vi "Manual Mode.vi"(5 "slider shoot":dbl, 7 "Shooter":T1, 8 "engage shoot":bool, 9 "Potent":dbl, 11 "Button 1":bool) -> ()   [LabVIEW 2012]
uses:
  <vilib>/Rock Robotics/WPI/Solenoid/WPI_SolenoidValue.ctl
  <vilib>/Rock Robotics/WPI/Joystick/WPI_JoystickGetSetRefNum.vi
  <vilib>/Rock Robotics/WPI/RobotDrive/WPI_RobotDriveArcadeDrive_Standard(NoSaturation).vi
  <vilib>/Rock Robotics/WPI/RobotDrive/WPI_RobotDriveGetSetRefNum.vi
  <vilib>/Rock Robotics/WPI/Solenoid/WPI_SolenoidSetEnum.vi
panel:
  out "theoretical angle":dbl
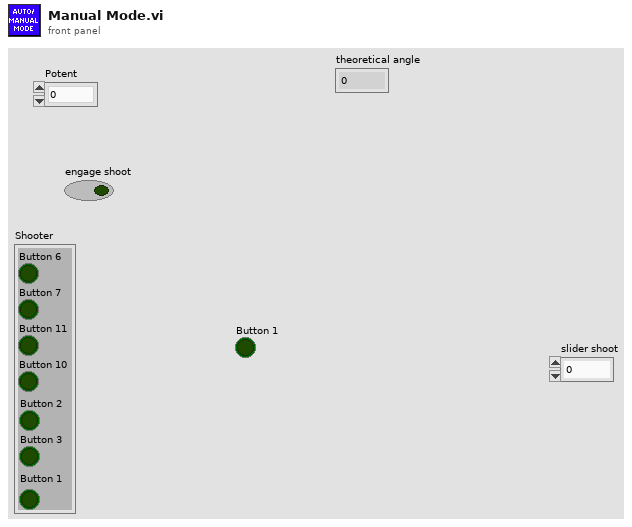
[diagram p1: front panel]
types:
  T1 = cluster{"Button 6":bool, "Button 7":bool, "Button 11":bool, "Button 10":bool, "Button 2":bool, "Button 3":bool, "Button 1":bool}
  T2 = typedef "WPI_JoystickDevRef.ctl" = cluster{"Device":T3}
  T3 = typedef "WPI_JoystickDeviceEnum.ctl" = enum16{"USB 1", "USB 2", "USB 3", "USB 4", "Kinect 1", "Kinect 2"}
  T4 = typedef "WPI_JoystickButtonState.ctl" = cluster{"Button 1":bool, "Button 2":bool, "Button 3":bool, "Button 4":bool, "Button 5":bool, "Button 6":bool, "Button 7":bool, "Button 8":bool, "Button 9":bool, "Button 10":bool, "Button 11":bool, "Button 12":bool}
  T5 = typedef "WPI_SolenoidDevRef.ctl" = cluster{"DevStatus":errorcluster, "Solenoid Module":T6, "Forward Solenoid Channel":T7, "Reverse Solenoid Channel":T7}
  T6 = typedef "FPGA_TypedefSolenoidModule.ctl" = enum16{"Solenoid Module 1", "Solenoid Module 2"}
  T7 = typedef "WPI_SolenoidChannel.ctl" = enum8{"Solenoid 1", "Solenoid 2", "Solenoid 3", "Solenoid 4", "Solenoid 5", "Solenoid 6", "Solenoid 7", "Solenoid 8", "Invalid"}
  T8 = typedef "WPI_MotorControlDeviceRef.ctl" = cluster{"DeviceStatus":errorcluster, "Type":enum16{"PWM", "CAN"}, "PWM":cluster{"Digital Module":T9, "PWM Channel":T10, "DeadBand":T11}, "CAN":cluster{"Device Number":u8, "Control Mode":T12, "Semaphore":T13, "Max Vout":dbl}, "Invert":bool, "TransformRef":T14, "InvTransformRef":T14}
  T9 = typedef "FPGA_TypedefDigitalModule.ctl" = enum16{"Digital Module 1", "Digital Module 2"}
  T10 = typedef "FPGA_DIOPWMChannel.ctl" = enum8{"PWM 1", "PWM 2", "PWM 3", "PWM 4", "PWM 5", "PWM 6", "PWM 7", "PWM 8", "PWM 9", "PWM 10", "Invalid"}
  T11 = typedef "WPI_PWMDeadband.ctl" = cluster{"Name":string, "maxPositivePwm":i32, "minPositivePwm":i32, "centerPwm":i32, "maxNegativePwm":i32, "minNegativePwm":i32, "angularRange":u16}
  T12 = typedef "WPI_CANJaguar_ControlMode.ctl" = enum8{"Percent VBus", "Current", "Speed", "Position", "Voltage"}
  T13 = typedef "Semaphore RefNum" = refnum<k1>
  T14 = typedef "WPI_PWMTransform_ConPane.ctl" = refnum<vi>
  T15 = typedef "WPI_SolenoidValue.ctl" = enum16{"Off", "On", "Forward", "Reverse"}
  T16 = typedef "WPI_RobotDriveDevRef.ctl" = cluster{"DevStatus":errorcluster, "Motors[]":T8[], "Square Inputs":bool, "Max Output":dbl, "Isochronous":bool}
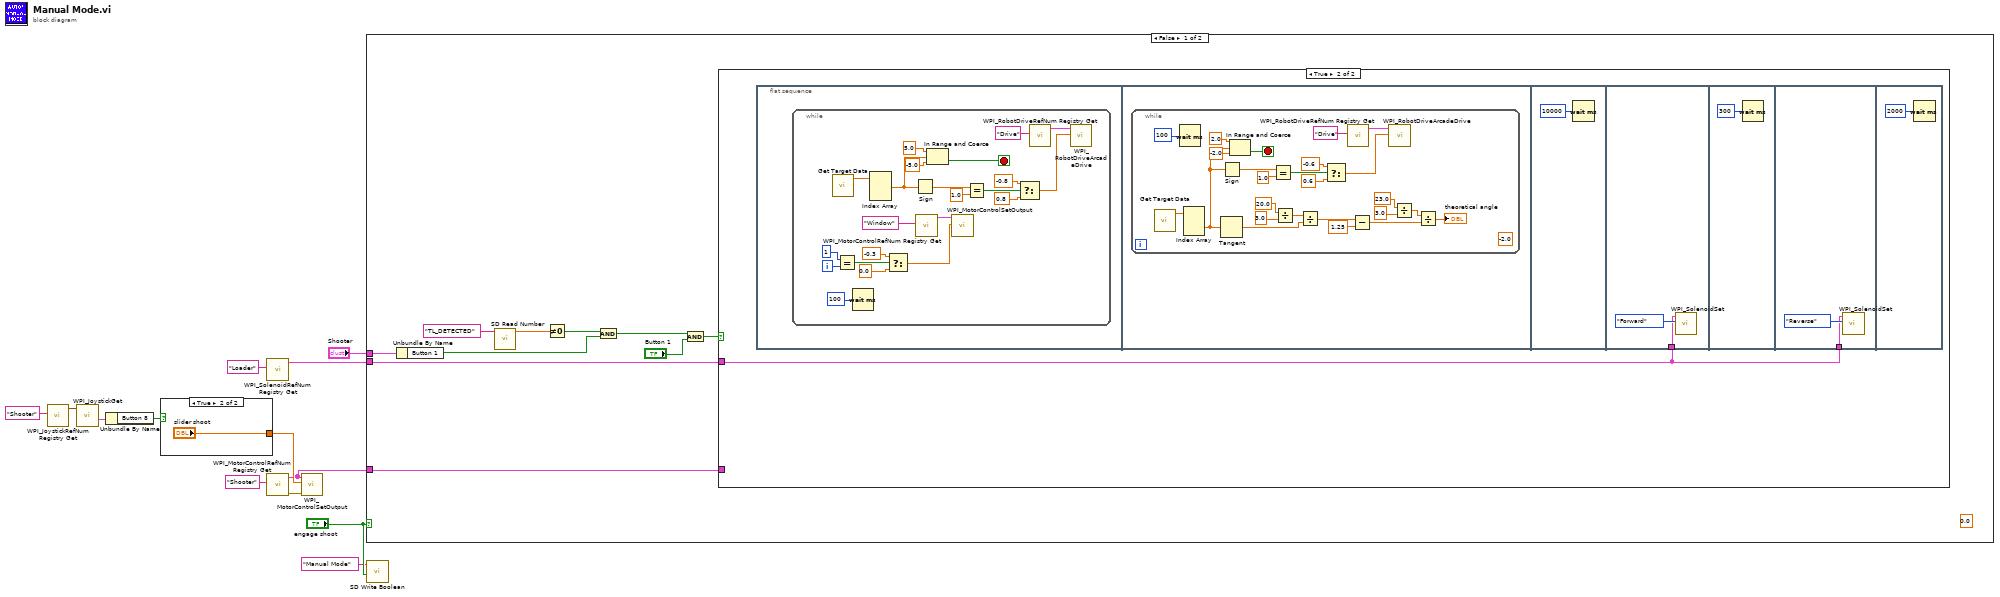
[diagram p0: block diagram]
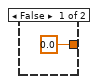
[diagram p2: hidden frame]
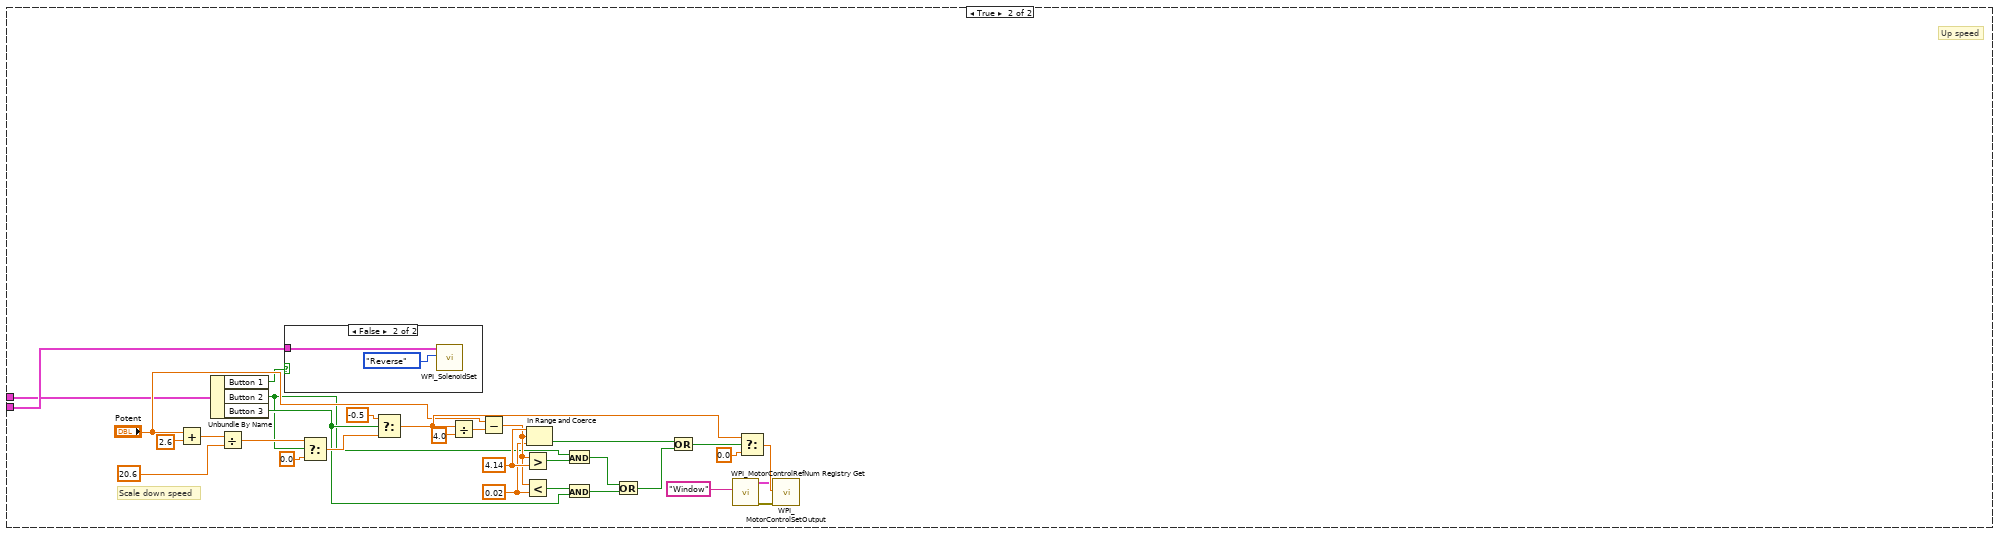
[diagram p4: hidden frame]
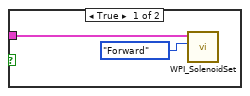
[diagram p5: hidden frame]
diagram:
  n1 = call <vilib>:"WPI_JoystickRefNum Registry Get.vi"("refnum name"="Shooter") -> ("JoystickDevRef"=w3:T2)  [unwired: 9 in, 1 out]
  n2 = call <vilib>:"WPI_JoystickGet.vi"("JoystickDevRef"=w3) -> ("Buttons"=w5:T4)  [unwired: 4 in, 2 out]
  n3 = Unbundle By Name(w5) -> ("Button 8"=w4:bool)
  n4 = case shown="True" w4 {
    tunnel: [0.0 ("slider shoot") "slider shoot"] -> w6
    frame False {
    }
    frame True {
    }
  }
  n5 = call <vilib>:"WPI_SolenoidRefNum Registry Get.vi"("refnum name"="Loader") -> ("SolenoidDevRef"=w11:T5)  [unwired: 9 in, 1 out]
  n6 = call <vilib>:"WPI_MotorControlRefNum Registry Get.vi"("refnum name"="Shooter") -> ("error out"=w8:errorcluster, "MotorControlDevRef"=w1:T8)  [unwired: 9 in]
  n7 = call <vilib>:"WPI_MotorControlSetOutput.vi"("error in (no error)"=w8, "Output"=w6, "MotorControlDevRef"=w1) -> ()  [unwired: 6 in, 3 out]
  n8 = case shown="False" "engage shoot" {
    tunnel: "Shooter" -> [w25 w81]
    tunnel: w11 -> [w22 w82]
    tunnel: w1 -> [w16 _]
    frame False {
      (unwired) 0.0 ("speed")
      n9 = Unbundle By Name(w25) -> ("Button 1"=w21:bool)
      n10 = call <vilib>:"SD Read Number.vi"("Name"="TL_DETECTED") -> ("Numeric"=w17:dbl)  [unwired: 8 in, 2 out]
      n11 = Not Equal To 0?(x=w17) -> (x != 0?=w18:bool)
      n12 = And(x=w18, y=w21) -> (x .and. y?=w20:bool)
      n13 = And(x=w20, y="Button 1") -> (x .and. y?=w24:bool)
      n14 = case shown="True" w24 {
        tunnel: w22 -> [_ w26]
        tunnel: w16 -> [_ _]
        frame False {
        }
        frame True {
          n15 = flat-sequence {
            tunnel: w26 -> [w75]
            tunnel: w26 -> [w78]
            frame #0 {
              n16 = while {
                i -> [w42]
                stop <- w27 stop-if-true
                n17 = call "Get Target Data.vi"() -> ("values"=w29:dbl[])  [unwired: 10 in, 1 out]
                n18 = Equal?(x=1, y=w42) -> (x = y?=w43:bool)
                n19 = Wait (ms)(milliseconds to wait=u32 100) -> ()  [unwired: 1 out]
                n20 = Index Array(array=w29) -> (element #1=w28:dbl)  [unwired: 3 in, 2 out]
                n21 = Select(t=-0.3, s=w43, f=0.0) -> (s? t:f=w40:dbl)
                n22 = Sign(1:w28) -> (0:w34:dbl)
                n23 = call <vilib>:"WPI_MotorControlRefNum Registry Get.vi"("refnum name"="Window") -> ("MotorControlDevRef"=w45:T8)  [unwired: 9 in, 1 out]
                n24 = In Range and Coerce(upper limit=5.0, x=w28, lower limit=-5.0) -> (In Range?=w27:bool)  [unwired: 1 out]
                n25 = call <vilib>:"WPI_MotorControlSetOutput.vi"("Output"=w40, "MotorControlDevRef"=w45) -> ()  [unwired: 7 in, 3 out]
                n26 = Equal?(x=w34, y=1.0) -> (x = y?=w33:bool)
                n27 = Select(t=-0.8, s=w33, f=0.8) -> (s? t:f=w30:dbl)
                n28 = call <vilib>:"WPI_RobotDriveRefNum Registry Get.vi"("refnum name"="Drive") -> ("RobotDriveDevRef"=w47:T16)  [unwired: 9 in, 1 out]
                n29 = call-poly <vilib>:"WPI_RobotDriveArcadeDrive.vi"("X axis value"=w30, "RobotDriveDevRef"=w47) -> ()  [unwired: 7 in, 3 out]
              }
            }
            frame #1 {
              n30 = while {
                stop <- w51 stop-if-true
                (unwired) -2.0 ("lower limit")
                n31 = call "Get Target Data.vi"() -> ("values"=w53:dbl[])  [unwired: 10 in, 1 out]
                n32 = Wait (ms)(milliseconds to wait=u32 100) -> ()  [unwired: 1 out]
                n33 = Index Array(array=w53) -> (element #2=w52:dbl)  [unwired: 3 in, 2 out]
                n34 = Sign(1:w52) -> (0:w56:dbl)
                n35 = Tangent(1:w52) -> (0:w63:dbl)
                n36 = In Range and Coerce(upper limit=2.0, x=w52, lower limit=-2.0) -> (In Range?=w51:bool)  [unwired: 1 out]
                n37 = Equal?(x=w56, y=1.0) -> (x = y?=w55:bool)
                n38 = Divide(x=20.0, y=3.0) -> (x/y=w70:dbl)
                n39 = Divide(x=w70, y=w63) -> (x/y=w64:dbl)
                n40 = Select(t=-0.6, s=w55, f=0.6) -> (s? t:f=w50:dbl)
                n41 = call <vilib>:"WPI_RobotDriveRefNum Registry Get.vi"("refnum name"="Drive") -> ("RobotDriveDevRef"=w72:T16)  [unwired: 9 in, 1 out]
                n42 = Subtract(x=w64, y=1.25) -> (x-y=w66:dbl)
                n43 = call-poly <vilib>:"WPI_RobotDriveArcadeDrive.vi"("X axis value"=w50, "RobotDriveDevRef"=w72) -> ()  [unwired: 7 in, 3 out]
                n44 = Divide(x=23.0, y=3.0) -> (x/y=w65:dbl)
                n45 = Divide(x=w65, y=w66) -> (x/y=→"theoretical angle":dbl)
              }
            }
            frame #2 {
              n46 = Wait (ms)(milliseconds to wait=u32 10000) -> ()  [unwired: 1 out]
            }
            frame #3 {
              n47 = call-poly <vilib>:"WPI_SolenoidSet.vi"("Value"=WPI_SolenoidValue."Forward", "SolenoidDevRef"=w75) -> ()  [unwired: 8 in, 2 out]
            }
            frame #4 {
              n48 = Wait (ms)(milliseconds to wait=u32 300) -> ()  [unwired: 1 out]
            }
            frame #5 {
              n49 = call-poly <vilib>:"WPI_SolenoidSet.vi"("Value"=WPI_SolenoidValue."Reverse", "SolenoidDevRef"=w78) -> ()  [unwired: 8 in, 2 out]
            }
            frame #6 {
              n50 = Wait (ms)(milliseconds to wait=u32 2000) -> ()  [unwired: 1 out]
            }
          }
        }
      }
    }
    frame True {
      w91 = 0.02 ("lower limit")
      w96 = 4.14 ("upper limit")
      # "Scale down speed"
      # "Up speed"
      n51 = Add(x="Potent", y=2.6) -> (x+y=w100:dbl)
      n52 = Unbundle By Name(w81) -> ("Button 1"=w83:bool, "Button 2"=w84:bool, "Button 3"=w85:bool)
      n53 = Divide(x=w100, y=20.6) -> (x/y=w97:dbl)
      n54 = case shown="False" w83 {
        tunnel: w82 -> [w112 w114]
        frame True {
          n55 = call-poly <vilib>:"WPI_SolenoidSet.vi"("Value"=WPI_SolenoidValue."Forward", "SolenoidDevRef"=w112) -> ()  [unwired: 8 in, 2 out]
        }
        frame False {
          n56 = call-poly <vilib>:"WPI_SolenoidSet.vi"("Value"=WPI_SolenoidValue."Reverse", "SolenoidDevRef"=w114) -> ()  [unwired: 8 in, 2 out]
        }
      }
      n57 = Select(t=w97, s=w84, f=0.0) -> (s? t:f=w95:dbl)
      n58 = Select(t=-0.5, s=w85, f=w95) -> (s? t:f=w104:dbl)
      n59 = Divide(x=w104, y=4.0) -> (x/y=w103:dbl)
      n60 = Subtract(x="Potent", y=w103) -> (x-y=w92:dbl)
      n61 = Greater?(x=w92, y=w96) -> (0:w94:bool)
      n62 = Less?(x=w92, y=w91) -> (x < y?=w90:bool)
      n63 = In Range and Coerce(upper limit=w96, x=w92, lower limit=w91) -> (In Range?=w86:bool)  [unwired: 1 out]
      n64 = And(x=w84, y=w94) -> (x .and. y?=w93:bool)
      n65 = And(x=w90, y=w85) -> (x .and. y?=w87:bool)
      n66 = Or(x=w93, y=w87) -> (x .or. y?=w89:bool)
      n67 = Or(x=w86, y=w89) -> (x .or. y?=w88:bool)
      n68 = call <vilib>:"WPI_MotorControlRefNum Registry Get.vi"("refnum name"="Window") -> ("error out"=w105:errorcluster, "MotorControlDevRef"=w106:T8)  [unwired: 9 in]
      n69 = Select(t=w104, s=w88, f=0.0) -> (s? t:f=w107:dbl)
      n70 = call <vilib>:"WPI_MotorControlSetOutput.vi"("error in (no error)"=w105, "Output"=w107, "MotorControlDevRef"=w106) -> ()  [unwired: 6 in, 3 out]
    }
  }
  n71 = call <vilib>:"SD Write Boolean.vi"("Boolean"="engage shoot", "Name"="Manual Mode") -> ()  [unwired: 8 in, 2 out]
